vi "ModeFieldOriented.vi"(1 "Drive Mode":T1(ring)) -> (0 "Orientation Mode":enum16{"Robot-Oriented", "Field-Oriented"}(ring))   [LabVIEW 2019]
doc: "This VI manages whether the swerve drive is in robot-oriented or field-oriented mode, based on driver inputs, emergency overrides, and safety interlocks."
uses:
  <vilib>/Rock Robotics/WPI/DriverStation/WPI_DriverStationRobotMode2.ctl
  dsinstructions.vi
  dsdata.vi
  sensors.vi
  outputs.vi
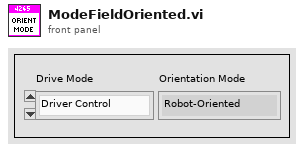
[diagram p1: front panel]
types:
  T1 = enum16{"Driver Control", "Auto Targeting", "Feeder Station"}
  T2 = typedef "WPI_DriverStationRobotMode2.ctl" = enum16{"Autonomous Disabled", "Autonomous Enabled", "Teleop Disabled", "Teleop Enabled", "Disconnected", "Finish", "Test Disabled", "Test Enabled", "Emergency Stopped"}
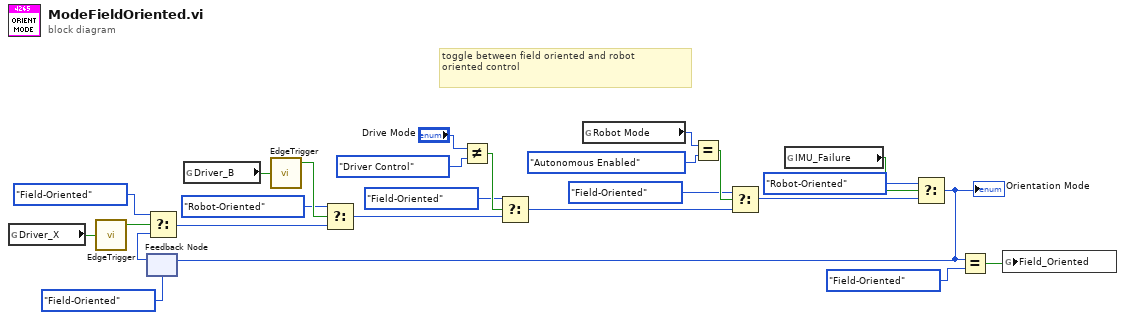
[diagram p0: block diagram]
diagram:
  # "toggle between field oriented and robot \noriented control"
  n1 = global read "dsinstructions.vi" "Driver_X"() -> (w19:bool)
  n2 = call "EdgeTrigger.vi"("Input Signal"=w19) -> ("Rising Edge Trigger"=w22:bool)  [unwired: 2 out]
  n3 = feedback #1(enum16{"Robot-Oriented", "Field-Oriented"}."Field-Oriented") -> (w21:enum16{"Robot-Oriented", "Field-Oriented"})
  n4 = Select(t=enum16{"Robot-Oriented", "Field-Oriented"}."Field-Oriented", s=w22, f=w21) -> (s? t:f=w20:enum16{"Robot-Oriented", "Field-Oriented"})
  n5 = global read "dsinstructions.vi" "Driver_B"() -> (w18:bool)
  n6 = call "EdgeTrigger.vi"("Input Signal"=w18) -> ("Rising Edge Trigger"=w16:bool)  [unwired: 2 out]
  n7 = Select(t=enum16{"Robot-Oriented", "Field-Oriented"}."Robot-Oriented", s=w16, f=w20) -> (s? t:f=w13:enum16{"Robot-Oriented", "Field-Oriented"})
  n8 = Not Equal?(x="Drive Mode", y=T1."Driver Control") -> (x != y?=w12:bool)
  n9 = Select(t=enum16{"Robot-Oriented", "Field-Oriented"}."Field-Oriented", s=w12, f=w13) -> (s? t:f=w11:enum16{"Robot-Oriented", "Field-Oriented"})
  n10 = global read "dsdata.vi" "Robot Mode"() -> (w23:T2)
  n11 = Equal?(x=w23, y=WPI_DriverStationRobotMode2."Autonomous Enabled") -> (x = y?=w25:bool)
  n12 = Select(t=enum16{"Robot-Oriented", "Field-Oriented"}."Field-Oriented", s=w25, f=w11) -> (s? t:f=w17:enum16{"Robot-Oriented", "Field-Oriented"})
  n13 = global read "sensors.vi" "IMU_Failure"() -> (w1:bool)
  n14 = Select(t=enum16{"Robot-Oriented", "Field-Oriented"}."Robot-Oriented", s=w1, f=w17) -> (s? t:f=w4:enum16{"Robot-Oriented", "Field-Oriented"})
  "Orientation Mode" <- w4
  n15 = feedback-in #1(w4) -> ()
  n16 = Equal?(x=w4, y=enum16{"Robot-Oriented", "Field-Oriented"}."Field-Oriented") -> (x = y?=w3:bool)
  n17 = global write "outputs.vi" "Field_Oriented"(w3) -> ()
